vi "Test Stop.vi"(11 "Error in":errorcluster) -> (15 "Error out":errorcluster)   [LabVIEW 2020, in "CelsiusToFarenheitTests.lvlib"]
doc: "This VI is to validate the stop button"
uses:
  CelsiusToFarenheitTests.lvlib
  <vilib>/SLL Drona/APIs/Assert/AssertVI/AssertVIExecRunning.vi
  <vilib>/SLL Drona/APIs/Stimulus/ControlValue/SetValueAuto.vi
  <vilib>/SLL Drona/APIs/Assert/AssertVI/AssertVIExecIdle.vi
  <vilib>/SLL Drona/APIs/Stimulus/VI/CloseVI.vi
  <vilib>/SLL Drona/Drona.lvlib
  <vilib>/addons/_JKI Toolkits/Caraya/classes/Test/Test.lvclass
  <vilib>/SLL Drona/APIs/Assert/AssertVI/AssertVI.lvlib
  <vilib>/SLL Drona/APIs/Stimulus/ControlValue/ControlValue.lvlib
  <vilib>/SLL Drona/APIs/Stimulus/VI/VI.lvlib
panel:
  # "STOP BUTTON TEST"
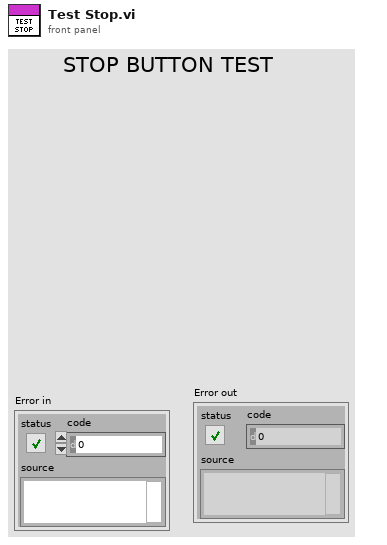
[diagram p1: front panel]
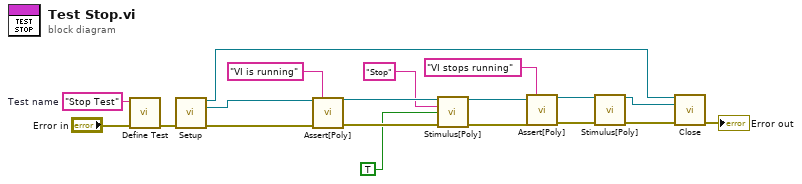
[diagram p0: block diagram]
diagram:
  w18 = "Stop Test"  # Test name
  n1 = call <vilib>:"Define Test.vi"("error in (no error)"="Error in", "Label (VI Title)"=w18) -> ("error out"=w19:errorcluster)  [unwired: 9 in]
  n2 = call <vilib>:"Setup.vi"("error in"=w19) -> ("Application Ref"=w17:refnum<vi>, "VI Reference Out"=w14:refnum<vi>, "error out"=w4:errorcluster)  [unwired: 12 in]
  n3 = call-poly <vilib>:"Assert[Poly].vi"("VI Reference In"=w14, "Test Label"="VI is running", "Error In"=w4) -> ("VI Reference Out"=w12:refnum<vi>, "Error Out"=w13:errorcluster)  [unwired: 11 in]
  n4 = call-poly <vilib>:"Stimulus[Poly].vi"("VI Reference In"=w12, "Control Path"="Stop", "Value (Signaling)"=TRUE, "error in"=w13) -> ("VI Reference Out"=w8:refnum<vi>, "error out"=w9:errorcluster)  [unwired: 10 in]
  n5 = call-poly <vilib>:"Assert[Poly].vi"("VI Reference In"=w8, "Test Label"="VI stops running", "Error In"=w9) -> ("VI Reference Out"=w5:refnum<vi>, "Error Out"=w6:errorcluster)  [unwired: 11 in]
  n6 = call-poly <vilib>:"Stimulus[Poly].vi"("VI Reference In"=w5, "error in"=w6) -> ("VI Reference Out"=w16:refnum<vi>, "error out"=w3:errorcluster)  [unwired: 12 in]
  n7 = call <vilib>:"Close.vi"("Application Ref"=w17, "VI Reference"=w16, "error in"=w3) -> ("error out"=→"Error out":errorcluster)  [unwired: 12 in]
